vi "Ver 1.0.vi"() -> ()   [LabVIEW 2015]
uses:
  <instrlib>/Keithley 2000/Keithley 2000.lvlib
  <instrlib>/Keithley 622x LV 2009/Keithley 622x.lvlib
  <instrlib>/Keithley 622x LV 2009/Utility/Typedefs/KE622x -- Instrument Type.ctl
  <instrlib>/Keithley 622x LV 2009/Configure/Source/Typedefs/KE622x -- Current Level.ctl
  <instrlib>/Keithley 622x LV 2009/Configure/Source/Typedefs/KE622x -- Voltage Limit.ctl
  <instrlib>/Keithley 2000/Public/Configure/Configure DC Volts.vi
  <instrlib>/Keithley 622x LV 2009/Configure/Source/Typedefs/KE622x -- Current Ranges.ctl
  <instrlib>/Keithley 622x LV 2009/Configure/Source/Typedefs/KE622x -- Current Range.ctl
  <instrlib>/Keithley 622x LV 2009/Typedefs/KE622x -- On Off Control.ctl
panel:
  in  "Custom Range (0 V) 2":dbl format="%#_6p"
  in  "Auto\nRange 2":bool
  out "ke2000 2":refnum<visa-resource-name>
  out "6221":refnum<visa-resource-name>
  in  "Floating-point file recording":bool
  in  "Comments":string
  in  "File name":string
  in  "Root Path":path=path "C:/"
  in  "Custom Range (0 V)":dbl format="%#_6p"
  in  "Step Level (A)":T1=0.01 min=-0.01 max=0.01 format="%.2p"
  in  "Stop Level (A)":T1=0.01 min=-0.01 max=0.01 format="%.2p"
  in  "Start Level (A)":T1=0.01 min=-0.01 max=0.01 format="%.2p"
  out "?":string
  out "?":string
  in  "Change Volt Ampers":bool
  out "fh":refnum<file>
  in  "Check For SCPI Errors? (T)":bool=TRUE
  out "Interlock Tripped?":bool
  out "Voltage Limit?":bool
  in  "Turn Off Output If Voltage Limit?":bool=TRUE
  in  "Output State":T2
  out "?":cluster{dbl[], dbl[]}[](graph)
  in  "Current Range In":T3={"Auto Range?"=TRUE, "Man / Selected\nRange"=enum."2nA"}
  in  "Voltage Limit (V) 3":T1=10.0 min=0.1 max=105.0 step=0.01 format="%.2p"
  out "ke6221":refnum<visa-resource-name>
  in  "Auto\nRange":bool
  in  "Interval (s)":dbl=1.0 min=1.0
  out "?":cluster{T1[], T1[]}(graph)
  out "ke2000":refnum<visa-resource-name>
  # "FILE CONFIGURATION"
  # "KE2000 Options"
  # "KE6221 Options"
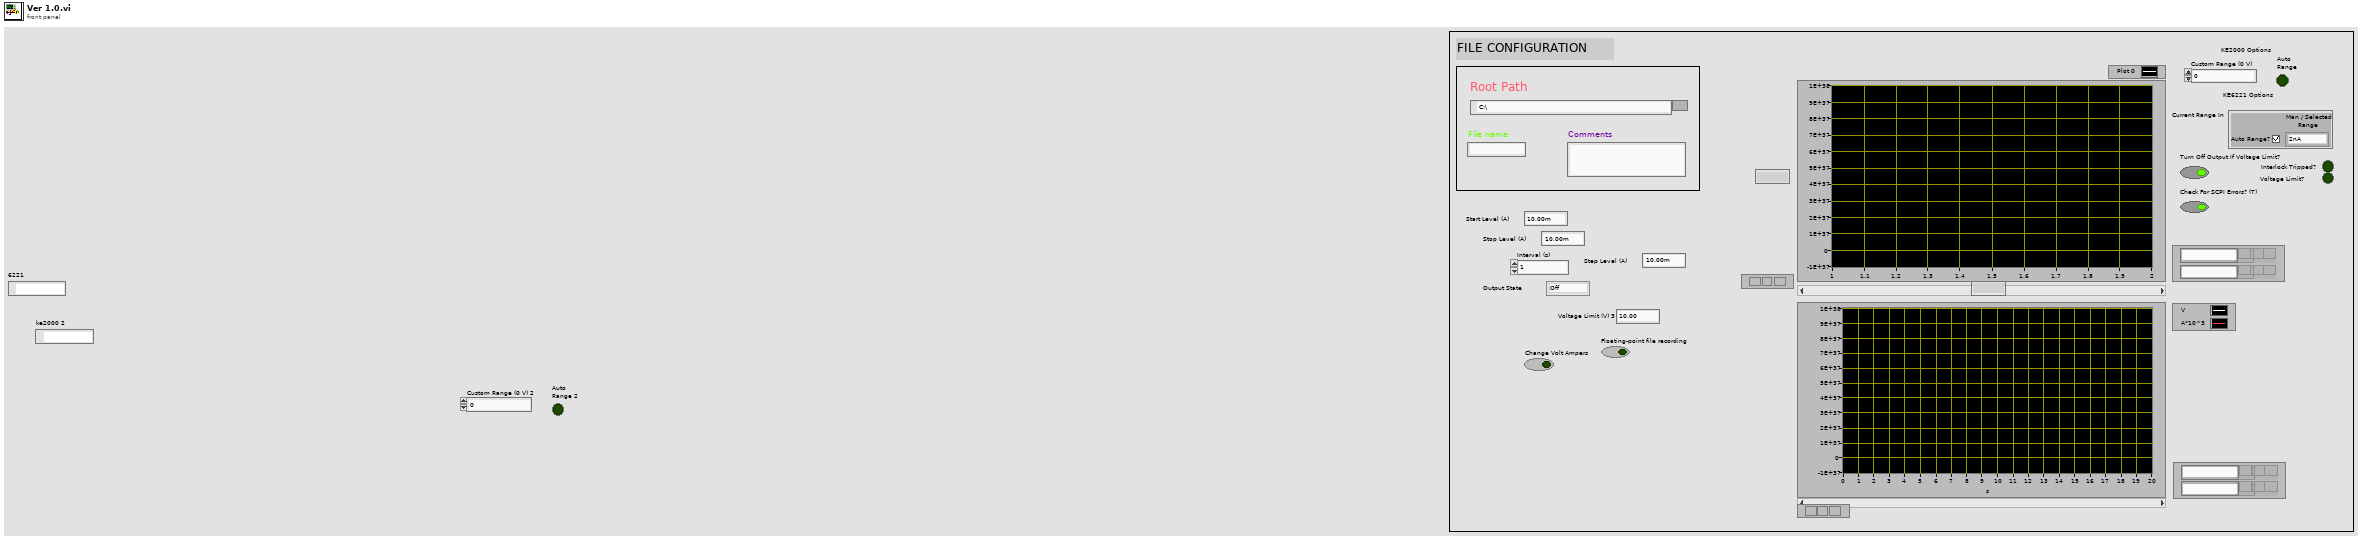
[diagram p1: front panel]
types:
  T1 = typedef "Keithley 622x.lvlib/KE622x -- Voltage Limit.ctl" = dbl
  T2 = typedef "Keithley 622x.lvlib/KE622x -- On Off Control.ctl" = enum16{"Off", "On"}
  T3 = typedef "Keithley 622x.lvlib/KE622x -- Current Range.ctl" = cluster{"Auto Range?":bool, "Man / Selected\nRange":T4}
  T4 = typedef "Keithley 622x.lvlib/KE622x -- Current Ranges.ctl" = enum16{"2nA", "20nA", "200nA", "2uA", "20uA", "200uA", "2mA", "20mA", "100mA"}
  T5 = typedef "Keithley 622x.lvlib/KE622x -- Instrument Type.ctl" = enum16{"KE6220", "KE6221"}
  T6 = enum16{"open", "replace", "create", "open or create", "replace or create", "replace or create with confirmation"}
  T7 = typedef "Keithley 622x.lvlib/KE622x -- Current Level.ctl" = dbl
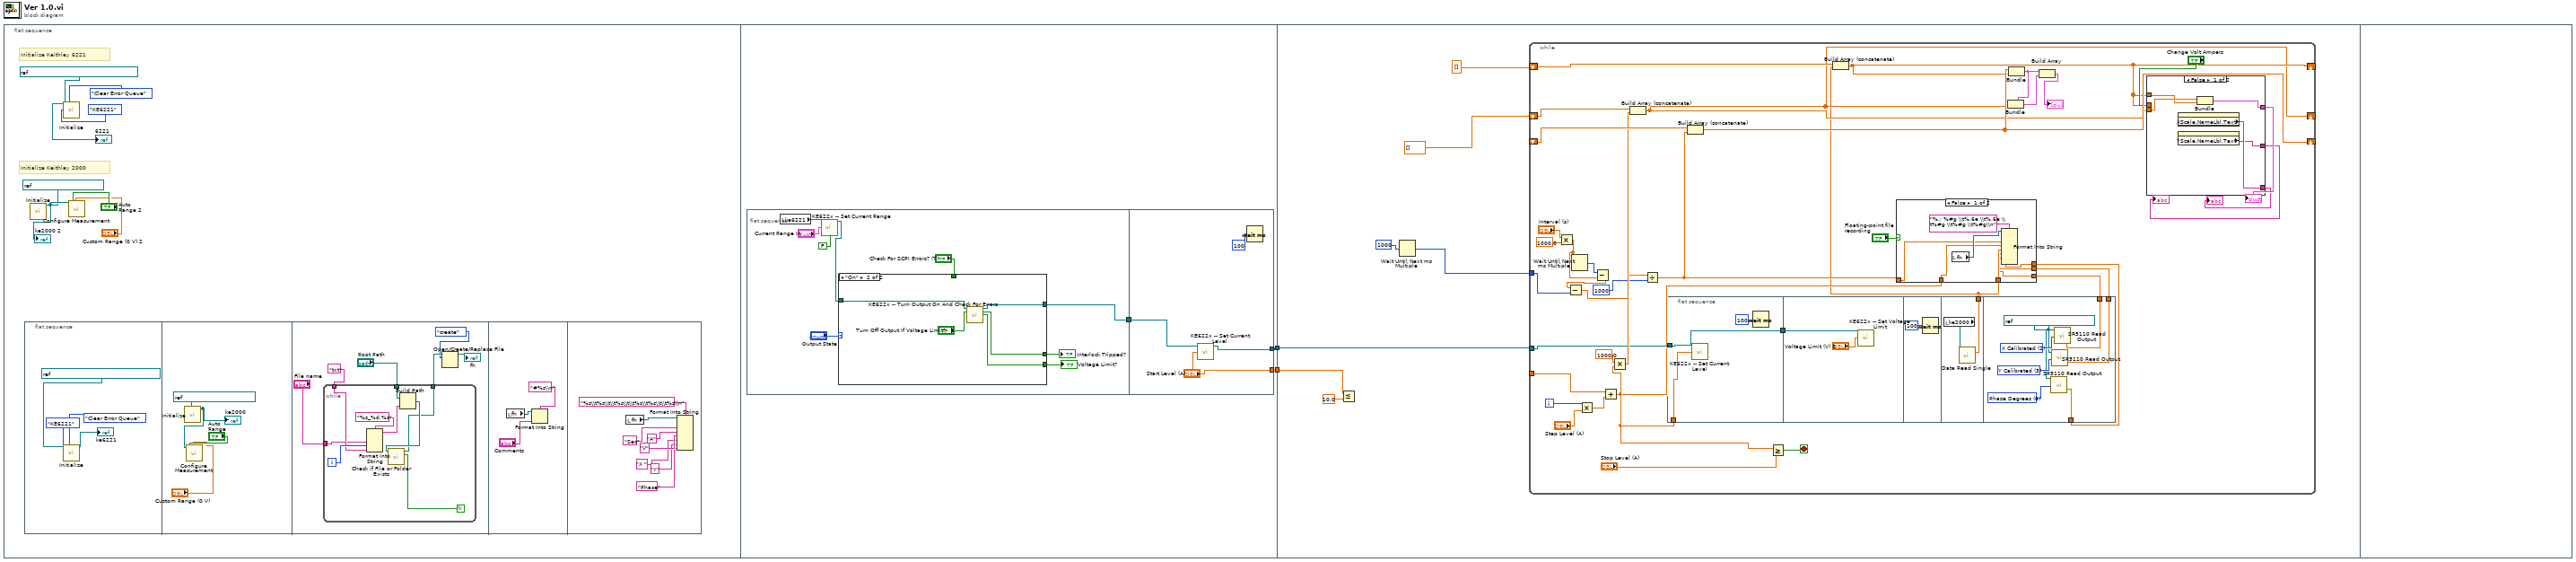
[diagram p0: block diagram]
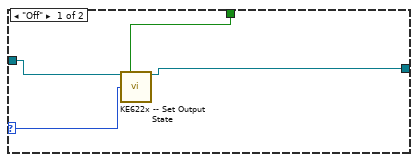
[diagram p2: hidden frame]
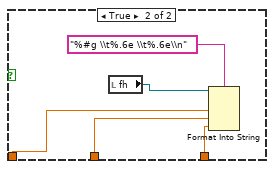
[diagram p3: hidden frame]
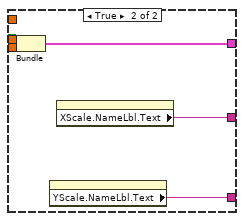
[diagram p4: hidden frame]
diagram:
  n1 = flat-sequence {
    tunnel: [w47] -> w2
    tunnel: [w46] -> w1
    tunnel: w2 -> [w72]
    tunnel: w1 -> [w74]
    frame #0 {
      # "Initialize Keithley 2000"
      # "Initialize Keithley 6221"
      n2 = flat-sequence {
        frame #0 {
          n3 = call <instrlib>:"Initialize.vi"("VISA resource name"=refnum<visa-resource-name> "KEITHLEY_DC_AC_CURRENT_SOURCE", "Error Queue Option"=enum16{"Clear Error Queue", "Error Query"}."Clear Error Queue", "Instrument Type"=KE622x_--_Instrument_Type."KE6221") -> ("VISA resource name out"=→"ke6221":refnum<visa-resource-name>)  [unwired: 11 in, 1 out]
        }
        frame #1 {
          n4 = call <instrlib>:"Initialize.vi"("VISA resource name"=refnum<visa-resource-name> "KEITHLEY_MULTIMETER") -> ("VISA resource name out"=w18:refnum<visa-resource-name>)  [unwired: 17 in, 1 out]
          "ke2000" <- w18
          n5 = call-poly <instrlib>:"Configure Measurement.vi"("VISA resource name"=w18, "Auto Range? (T: Auto)"="Auto\nRange", "Custom Range (0 V)"="Custom Range (0 V)") -> ()  [unwired: 15 in, 2 out]
        }
        frame #2 {
          n6 = while {
            tunnel: "txt" ("format string") -> [w31]
            tunnel: "File name" -> [w30]
            tunnel: "Root Path" -> [w28]
            tunnel: [w26] -> w21
            i -> [w32]
            stop <- w25 continue-if-true
            n7 = Format Into String(format string="%s_%d.%s", w30, w32, w31) -> (resulting string=w29:string)  [unwired: 2 in, 1 out]
            n8 = Build Path(base path=w28, name or relative path=w29) -> (appended path=w27:path)
            n9 = call <vilib>:"Check if File or Folder Exists.vi"("path"=w27) -> ("file or folder exists?"=w25:bool, "dup path"=w26:path)  [unwired: 8 in, 1 out]
          }
          n10 = Open/Create/Replace File(file path (use dialog)=w21, operation (0:open)=T6."create") -> (refnum out=→"fh":refnum<file>)  [unwired: 4 in, 2 out]
        }
        frame #3 {
          n11 = local read "fh"() -> (w36:refnum<file>)
          n12 = Format Into String(format string="#%s\\n", initial string=w36, "Comments") -> ()  [unwired: 1 in, 2 out]
        }
        frame #4 {
          n13 = local read "fh"() -> (w44:refnum<file>)
          n14 = Format Into String(format string="%s\\t%s\\t\\t%s\\t\\t%s\\t%s\\t\\t%s\\n", initial string=w44, "Sec" ("input 1"), "A" ("input 2"), "V" ("input 3"), "X " ("input 3"), "Y" ("input 3"), "Phase" ("input 3")) -> ()  [unwired: 1 in, 2 out]
        }
      }
      n15 = call <instrlib>:"Initialize.vi"("VISA resource name"=refnum<visa-resource-name> "KEITHLEY_MULTIMETER") -> ("VISA resource name out"=w6:refnum<visa-resource-name>)  [unwired: 17 in, 1 out]
      "ke2000 2" <- w6
      n16 = call <instrlib>:"Initialize.vi"("VISA resource name"=refnum<visa-resource-name> "KEITHLEY_DC_AC_CURRENT_SOURCE", "Error Queue Option"=enum16{"Clear Error Queue", "Error Query"}."Clear Error Queue", "Instrument Type"=KE622x_--_Instrument_Type."KE6221") -> ("VISA resource name out"=→"6221":refnum<visa-resource-name>)  [unwired: 11 in, 1 out]
      n17 = call-poly <instrlib>:"Configure Measurement.vi"("VISA resource name"=w6, "Auto Range? (T: Auto)"="Auto\nRange 2", "Custom Range (0 V)"="Custom Range (0 V) 2") -> ()  [unwired: 15 in, 2 out]
    }
    frame #1 {
      n18 = flat-sequence {
        tunnel: [w48] -> w45
        tunnel: ["Start Level (A)"] -> w47
        tunnel: [w67] -> w46
        tunnel: w45 -> [w66]
        frame #0 {
          n19 = local read "ke6221"() -> (w51:refnum<visa-resource-name>)
          n20 = call <instrlib>:"KE622x -- Set Current Range.vi"("Resource In"=w51, "Current Range In"="Current Range In", "Read Back Set Values? (T)"=FALSE) -> ("Resource Out (dupl)"=w56:refnum<visa-resource-name>)  [unwired: 10 in, 2 out]
          n21 = case shown="\"On\"" "Output State" {
            selector: "Output State" -> [w60 _]
            tunnel: [_ w64] -> w54
            tunnel: [_ w63] -> w55
            tunnel: "Check For SCPI Errors? (T)" -> [w59 _]
            tunnel: w56 -> [w57 w62]
            tunnel: [w58 w61] -> w48
            frame "Off" {
              n22 = call <instrlib>:"KE622x -- Set Output State.vi"("Resource In"=w57, "Check For SCPI Errors? (T)"=w59, "Output State"=w60) -> ("Resource Out (dupl)"=w58:refnum<visa-resource-name>)  [unwired: 11 in, 1 out]
            }
            frame "On" {
              n23 = call <instrlib>:"KE622x -- Turn Output On And Check For Errors.vi"("Resource In"=w62, "Turn Off Output If Compliance?"="Turn Off Output If Voltage Limit?") -> ("Resource Out (dupl)"=w61:refnum<visa-resource-name>, "Interlock Tripped?"=w64:bool, "Compliance?"=w63:bool)  [unwired: 10 in, 1 out]
            }
          }
          "Interlock Tripped?" <- w54
          "Voltage Limit?" <- w55
        }
        frame #1 {
          n24 = call <instrlib>:"KE622x -- Set Current Level.vi"("Resource In"=w66, "Current Level (A) In"="Start Level (A)") -> ("Resource Out (dupl)"=w67:refnum<visa-resource-name>)  [unwired: 12 in, 1 out]
          n25 = Wait (ms)(milliseconds to wait=u32 100) -> ()  [unwired: 1 out]
        }
      }
    }
    frame #2 {
      n26 = Less Or Equal?(x=w72, y=T1 10.0) -> (x <= y?=w73:bool)
      n27 = Wait Until Next ms Multiple(millisecond multiple=u32 1000) -> (millisecond timer value=w75:u32)
      n28 = while {
        shift-right: [w107] -> _
        shift-left: dbl[] [] -> [w116]
        shift-right: [w112] -> _
        shift-left: _ -> [w114]
        shift-right: [w99] -> _
        shift-left: T7[] [] -> [w113]
        tunnel: w74 -> [w92]
        tunnel: [w91] -> w70
        tunnel: w75 -> [w86]
        i -> [w104]
        stop <- w101 stop-if-true
        n29 = Multiply(x="Interval (s)", y=1000.0) -> (x*y=w87:dbl)
        n30 = Wait Until Next ms Multiple(millisecond multiple=w87) -> (millisecond timer value=w90:u32)
        n31 = Multiply(x=w104, y="Step Level (A)") -> (x*y=w103:T1)
        n32 = Subtract(x=w90, y=w87) -> (x-y=w85:dbl)
        n33 = Subtract(x=w85, y=w86) -> (x-y=w84:dbl)
        n34 = Add(x=w91, y=w103) -> (x+y=w88:T1)
        n35 = Multiply(x=T1 1000.0, y=w88) -> (x*y=w98:T1)
        n36 = Build Array (concatenate)(w113, w98) -> (w99:T1[])
        n37 = Divide(x=w84, y=1000) -> (x/y=w95:dbl)
        n38 = flat-sequence {
          tunnel: w88 -> [w133]
          tunnel: w92 -> [w132]
          tunnel: [w131] -> w89
          tunnel: w89 -> [w134]
          tunnel: [w137] -> w81
          tunnel: [w145] -> w82
          tunnel: [w140] -> w80
          tunnel: [w139] -> w79
          frame #0 {
            n39 = call <instrlib>:"KE622x -- Set Current Level.vi"("Resource In"=w132, "Current Level (A) In"=w133) -> ("Resource Out (dupl)"=w131:refnum<visa-resource-name>)  [unwired: 12 in, 1 out]
            n40 = Wait (ms)(milliseconds to wait=u32 100) -> ()  [unwired: 1 out]
          }
          frame #1 {
            n41 = call <instrlib>:"KE622x -- Set Voltage Limit.vi"("Resource In"=w134, "Voltage Limit (V)"="Voltage Limit (V) 3") -> ()  [unwired: 12 in, 2 out]
          }
          frame #2 {
            n42 = Wait (ms)(milliseconds to wait=u32 100) -> ()  [unwired: 1 out]
          }
          frame #3 {
            n43 = local read "ke2000"() -> (w138:refnum<visa-resource-name>)
            n44 = call <instrlib>:"Data Read Single.vi"("VISA resource name"=w138) -> ("Measurement"=w137:dbl)  [unwired: 14 in, 4 out]
          }
          frame #4 {
            w142 = u16 6 items=["X %", "Y %", "X Calibrated", "Y Calibrated", "Mag %", "Mag Calibrated", "Phase Degrees", "Ratio", "ADC 1", "ADC 2", "ADC 3", "ADC 4 ", "Noise %", "Noise Calibrated", "Ref Frequency", "", ""] ("Display Type")
            w143 = u16 3 items=["X %", "Y %", "X Calibrated", "Y Calibrated", "Mag %", "Mag Calibrated", "Phase Degrees", "Ratio", "ADC 1", "ADC 2", "ADC 3", "ADC 4 ", "Noise %", "Noise Calibrated", "Ref Frequency", "", ""] ("Display Type")
            w144 = u16 2 items=["X %", "Y %", "X Calibrated", "Y Calibrated", "Mag %", "Mag Calibrated", "Phase Degrees", "Ratio", "ADC 1", "ADC 2", "ADC 3", "ADC 4 ", "Noise %", "Noise Calibrated", "Ref Frequency", "", ""] ("Display Type")
            w141 = refnum<visa-resource-name> "LOCK_IN_5110_PRINCETON" ("VISA session (for class)")
            n45 = call "SR5110 Read Output"("VISA session (for class)"=w141, "Display Type"=w142) -> ("Output (FP)"=w139:dbl)  [unwired: 9 in, 8 out]
            n46 = call "SR5110 Read Output"("VISA session (for class)"=w141, "Display Type"=w143) -> ("Output (FP)"=w140:dbl)  [unwired: 9 in, 8 out]
            n47 = call "SR5110 Read Output"("VISA session (for class)"=w141, "Display Type"=w144) -> ("Display"=w145:dbl)  [unwired: 9 in, 8 out]
          }
        }
        n48 = Build Array (concatenate)(w114, w95) -> (w112:dbl[])
        n49 = Greater Or Equal?(x=w88, y="Stop Level (A)") -> (x >= y?=w101:bool)
        n50 = Build Array (concatenate)(w116, w81) -> (w107:dbl[])
        n51 = case shown="False" "Floating-point file recording" {
          tunnel: w95 -> [w120 w127]
          tunnel: w81 -> [w122 w126]
          tunnel: w88 -> [w121 w125]
          tunnel: w82 -> [w119 _]
          tunnel: w80 -> [w118 _]
          tunnel: w79 -> [w117 _]
          frame False {
            n52 = local read "fh"() -> (w123:refnum<file>)
            n53 = Format Into String(format string="%.; %#g \\t%.6e \\t%.6e \\t%#g \\t%#g \\t%#g\\n", initial string=w123, w120, w121, w122, w119, w118, w117) -> ()  [unwired: 1 in, 2 out]
          }
          frame True {
            n54 = local read "fh"() -> (w128:refnum<file>)
            n55 = Format Into String(format string="%#g \\t%.6e \\t%.6e\\n", initial string=w128, w127, w125, w126) -> ()  [unwired: 1 in, 2 out]
          }
        }
        n56 = Bundle(w112, w107) -> (w110:cluster{dbl[], dbl[]})  [unwired: 1 in]
        n57 = Bundle(cluster=w110, w99) -> (w111:cluster{dbl[], dbl[]})  [unwired: 1 in]
        n58 = Build Array(w110, w111) -> (→"?":cluster{dbl[], dbl[]}[])
        n59 = case shown="False" "Change Volt Ampers" {
          tunnel: [w150 w155] -> w115
          tunnel: w107 -> [_ w154]
          tunnel: w99 -> [w149 w153]
          tunnel: w107 -> [w148 _]
          tunnel: [w146 w152] -> w106
          tunnel: [w147 w151] -> w105
          frame False {
            n60 = property class="XYGraph (strict)"() -> ("YScale.NameLbl.Text"=w146:string)  [unwired: 2 in, 2 out]
            n61 = property class="XYGraph (strict)"() -> ("XScale.NameLbl.Text"=w147:string)  [unwired: 2 in, 2 out]
            n62 = Bundle(w149, w148) -> (w150:cluster{T1[], dbl[]})  [unwired: 1 in]
          }
          frame True {
            n63 = Bundle(w154, w153) -> (w155:cluster{dbl[], T1[]})  [unwired: 1 in]
            n64 = property class="XYGraph (strict)"() -> ("YScale.NameLbl.Text"=w151:string)  [unwired: 2 in, 2 out]
            n65 = property class="XYGraph (strict)"() -> ("XScale.NameLbl.Text"=w152:string)  [unwired: 2 in, 2 out]
          }
        }
        "?" <- w115
        "?" <- w106
        "?" <- w105
      }
    }
    frame #3 {
    }
  }
